vi "Remove Director.vi"(8 "error in (no error)":errorcluster, 10 "Command Director Id":string, 11 "InteractionProcessor in":refnum<class "InteractionProcessor.lvclass">) -> (0 "error out":errorcluster, 2 "Command Director Removed":refnum<class "CommandDirector.lvclass">, 3 "InteractionProcessor out":refnum<class "InteractionProcessor.lvclass">)   [LabVIEW 2023, in "HAF.lvlib" / "InteractionProcessor.lvclass"]
uses:
  InteractionProcessor.lvclass
  CommandDirector/CommandDirector.lvclass
panel:
  out "Removed?":bool
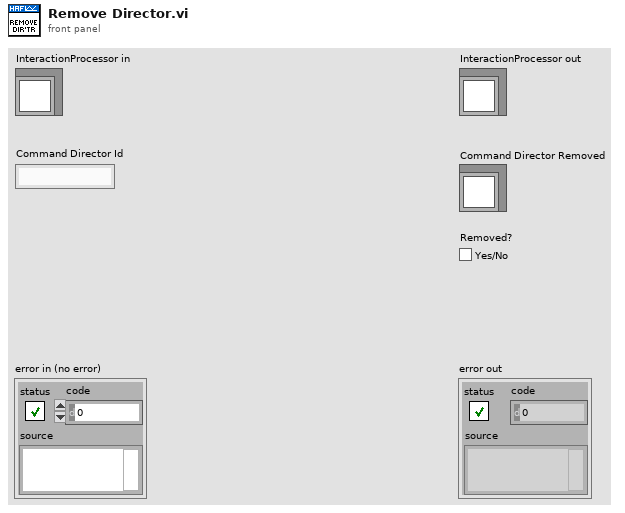
[diagram p1: front panel]
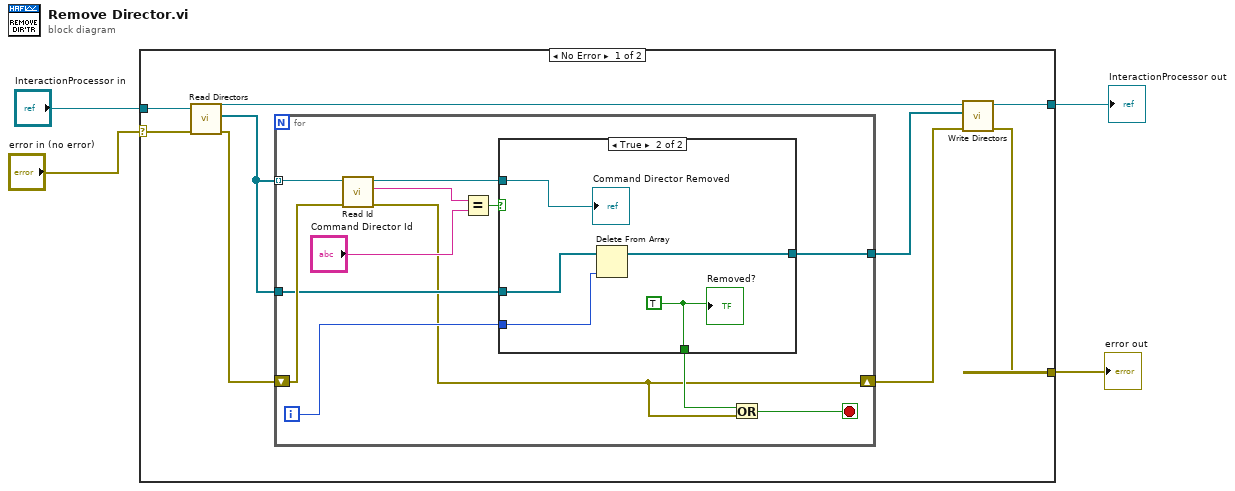
[diagram p0: block diagram]
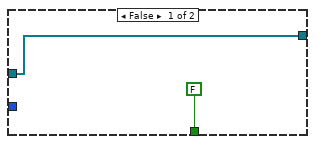
[diagram p2: hidden frame]
diagram:
  n1 = case shown="No Error" "error in (no error)" {
    selector: "error in (no error)" -> [w12 w34]
    tunnel: [w5 w34] -> w3
    tunnel: [w11 w33] -> w1
    tunnel: "InteractionProcessor in" -> [w13 w33]
    frame No Error {
      n2 = call-dynamic "Read Directors.vi"("error in (no error)"=w12, "InteractionProcessor in"=w13) -> ("error out"=w9:errorcluster, "Directors"=w10:refnum<class "CommandDirector.lvclass">[], "InteractionProcessor out"=w7:refnum<class "InteractionProcessor.lvclass">)  [unwired: 7 in]
      n3 = for {
        tunnel: w10 -> [w25] mode=indexing
        tunnel: w10 -> [w19]
        shift-right: [w14] -> w8
        shift-left: w9 -> [w24]
        tunnel: [w17] -> w6
        i -> [w18]
        stop <- w16 stop-if-true
        n4 = call-dynamic "Read Id.vi"("error in (no error)"=w24, "CommandDirector in"=w25) -> ("error out"=w14:errorcluster, "Id"=w23:string, "CommandDirector out"=w21:refnum<class "CommandDirector.lvclass">)  [unwired: 7 in]
        n5 = Equal?(x=w23, y="Command Director Id") -> (x = y?=w20:bool)
        n6 = case shown="True" w20 {
          tunnel: w21 -> [_ w32]
          tunnel: w19 -> [w27 w31]
          tunnel: w18 -> [_ w30]
          tunnel: [w27 w29] -> w17
          tunnel: [FALSE w28] -> w15
          frame False {
          }
          frame True {
            w28 = TRUE
            n7 = Delete From Array(array=w31, index=w30) -> (array with subset deleted=w29:refnum<class "CommandDirector.lvclass">[])  [unwired: 1 in, 1 out]
            "Command Director Removed" <- w32
            "Removed?" <- w28
          }
        }
        n8 = Or(x=w15, y=w14) -> (x .or. y?=w16:bool)
      }
      n9 = call-dynamic "Write Directors.vi"("error in (no error)"=w8, "Directors"=w6, "InteractionProcessor in"=w7) -> ("error out"=w5:errorcluster, "InteractionProcessor out"=w11:refnum<class "InteractionProcessor.lvclass">)  [unwired: 7 in]
    }
    frame Error {
    }
  }
  "error out" <- w3
  "InteractionProcessor out" <- w1
